vi "Modify Target with timeout (SubVI).vi"(4 "Max Rate":dbl, 6 "Default Rate":dbl, 7 "Target in":dbl, 9 "Sweep rate in":dbl, 10 "Timeout (s) in":u16, 11 "Present value":dbl) -> (1 "Timeout (s) out":dbl, 2 "Sweep rate out":dbl, 3 "Target out":dbl)   [LabVIEW 2025, in "Cryo.lvlib"]
uses:
  Cryo.lvlib
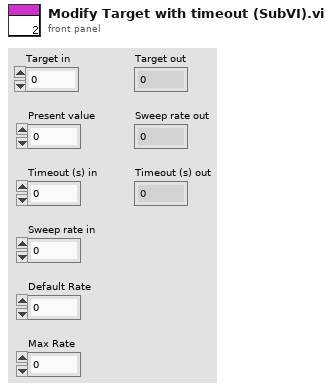
[diagram p1: front panel]
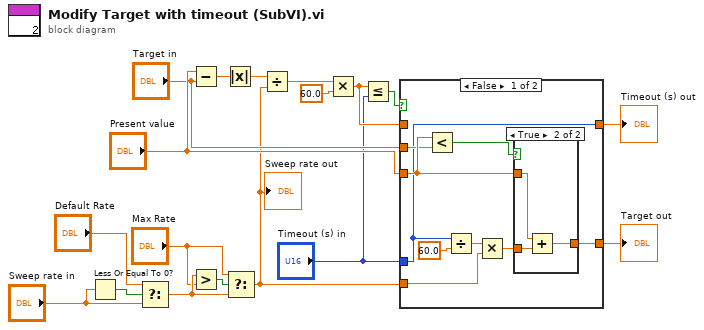
[diagram p0: block diagram]
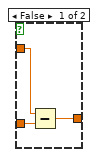
[diagram p2: hidden frame]
diagram:
  n1 = Less Or Equal To 0?(x="Sweep rate in") -> (x <= 0?=w5:bool)
  n2 = Select(t="Default Rate", s=w5, f="Sweep rate in") -> (s? t:f=w8:dbl)
  n3 = Subtract(x="Present value", y="Target in") -> (x-y=w14:dbl)
  n4 = Greater?(x=w8, y="Max Rate") -> (0:w6:bool)
  n5 = Absolute Value(x=w14) -> (abs(x)=w3:dbl)
  n6 = Select(t="Max Rate", s=w6, f=w8) -> (s? t:f=w13:dbl)
  "Sweep rate out" <- w13
  n7 = Divide(x=w3, y=w13) -> (x/y=w1:dbl)
  n8 = Multiply(x=w1, y=60.0) -> (x*y=w16:dbl)
  n9 = Less Or Equal?(x=w16, y="Timeout (s) in") -> (x <= y?=w10:bool)
  n10 = case shown="False" w10 {
    tunnel: "Target in" -> [w21 w35]
    tunnel: [w20 w35] -> w11
    tunnel: [w19 w34] -> w18
    tunnel: "Timeout (s) in" -> [w19 _]
    tunnel: w13 -> [w25 _]
    tunnel: "Present value" -> [w22 _]
    tunnel: w16 -> [_ w34]
    frame False {
      n11 = Less?(x=w22, y=w21) -> (x < y?=w23:bool)
      n12 = Divide(x=w19, y=60.0) -> (x/y=w26:dbl)
      n13 = Multiply(x=w26, y=w25) -> (x*y=w24:dbl)
      n14 = case shown="True" w23 {
        tunnel: w24 -> [w28 w32]
        tunnel: w22 -> [w29 w31]
        tunnel: [w30 w33] -> w20
        frame False {
          n15 = Subtract(x=w29, y=w28) -> (x-y=w30:dbl)
        }
        frame True {
          n16 = Add(x=w31, y=w32) -> (x+y=w33:dbl)
        }
      }
    }
    frame True {
    }
  }
  "Timeout (s) out" <- w18
  "Target out" <- w11
